vi "read station LIN config - 1.vi"(8 "error in":errorcluster, 10 "station idx":i32, 11 "configuration file path in":path) -> (0 "error out":errorcluster, 1 "LIN Device":T1={"Master Frame(3C)"="MasterReq\nSPA3414_ConfigurationsCMAGeely_CEMCALYPSOSDB34XX0Cfg_LIN3_190709_", "Slave Frame(3D)"="SlaveResp\nSPA3414_ConfigurationsCMAGeely_CEMCALYPSOSDB34XX0Cfg_LIN3_190709_", "Request Schedule"="CEMLIN3DiagRequestSchedule\nSPA3414_ConfigurationsCMAGeely_CEMCALYPSOSDB34XX0Cfg_LIN3_190709_", "Response Schedule"="CEMLIN3DiagResponseSchedule\nSPA3414_ConfigurationsCMAGeely_CEMCALYPSOSDB34XX0Cfg_LIN3_190709_", "Frame Write SCU"="", "Frame Read SCU"="", "LIN Name"=""}, 2 "LIN Device Name":string, 3 "configuration file path out":path)   [LabVIEW 2018]
uses:
  03.Inalfa LIN/LIN Device.ctl
  05.UserVI's/file io/ini/type defs/ini file actions.ctl
  05.UserVI's/file io/ini/type defs/ini entry value.ctl
  05.UserVI's/file io/ini/type defs/ini entry types.ctl
  05.UserVI's/file io/ini/type defs/ini entry.ctl
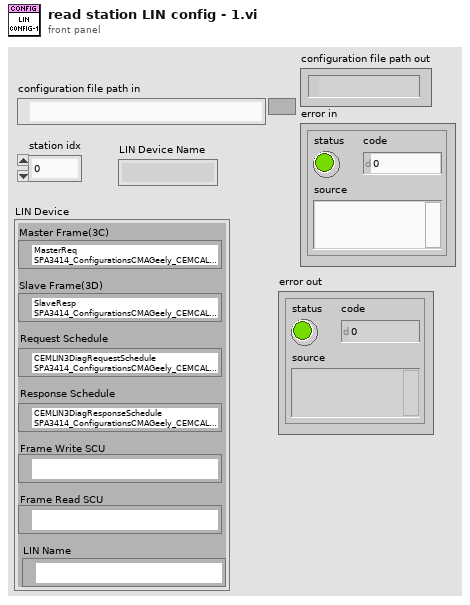
[diagram p1: front panel]
types:
  T1 = typedef "LIN Device.ctl" = cluster{"Master Frame(3C)":refnum<k21>, "Slave Frame(3D)":refnum<k21>, "Request Schedule":refnum<k21>, "Response Schedule":refnum<k21>, "Frame Write SCU":refnum<k21>, "Frame Read SCU":refnum<k21>, "LIN Name":refnum<k21>}
  T2 = typedef "ini entry value.ctl" = cluster{"Boolean":bool, "Dbl":dbl, "I32":i32, "Path":path, "String":string, "U32":u32}
  T3 = typedef "ini file actions.ctl" = enum16{"read ini", "write ini"}
  T4 = typedef "ini entry.ctl" = cluster{"section":string, "key":string, "type":T5, "default value":T2}
  T5 = typedef "ini entry types.ctl" = enum16{"Boolean", "Double", "I32", "Path", "String", "U32"}
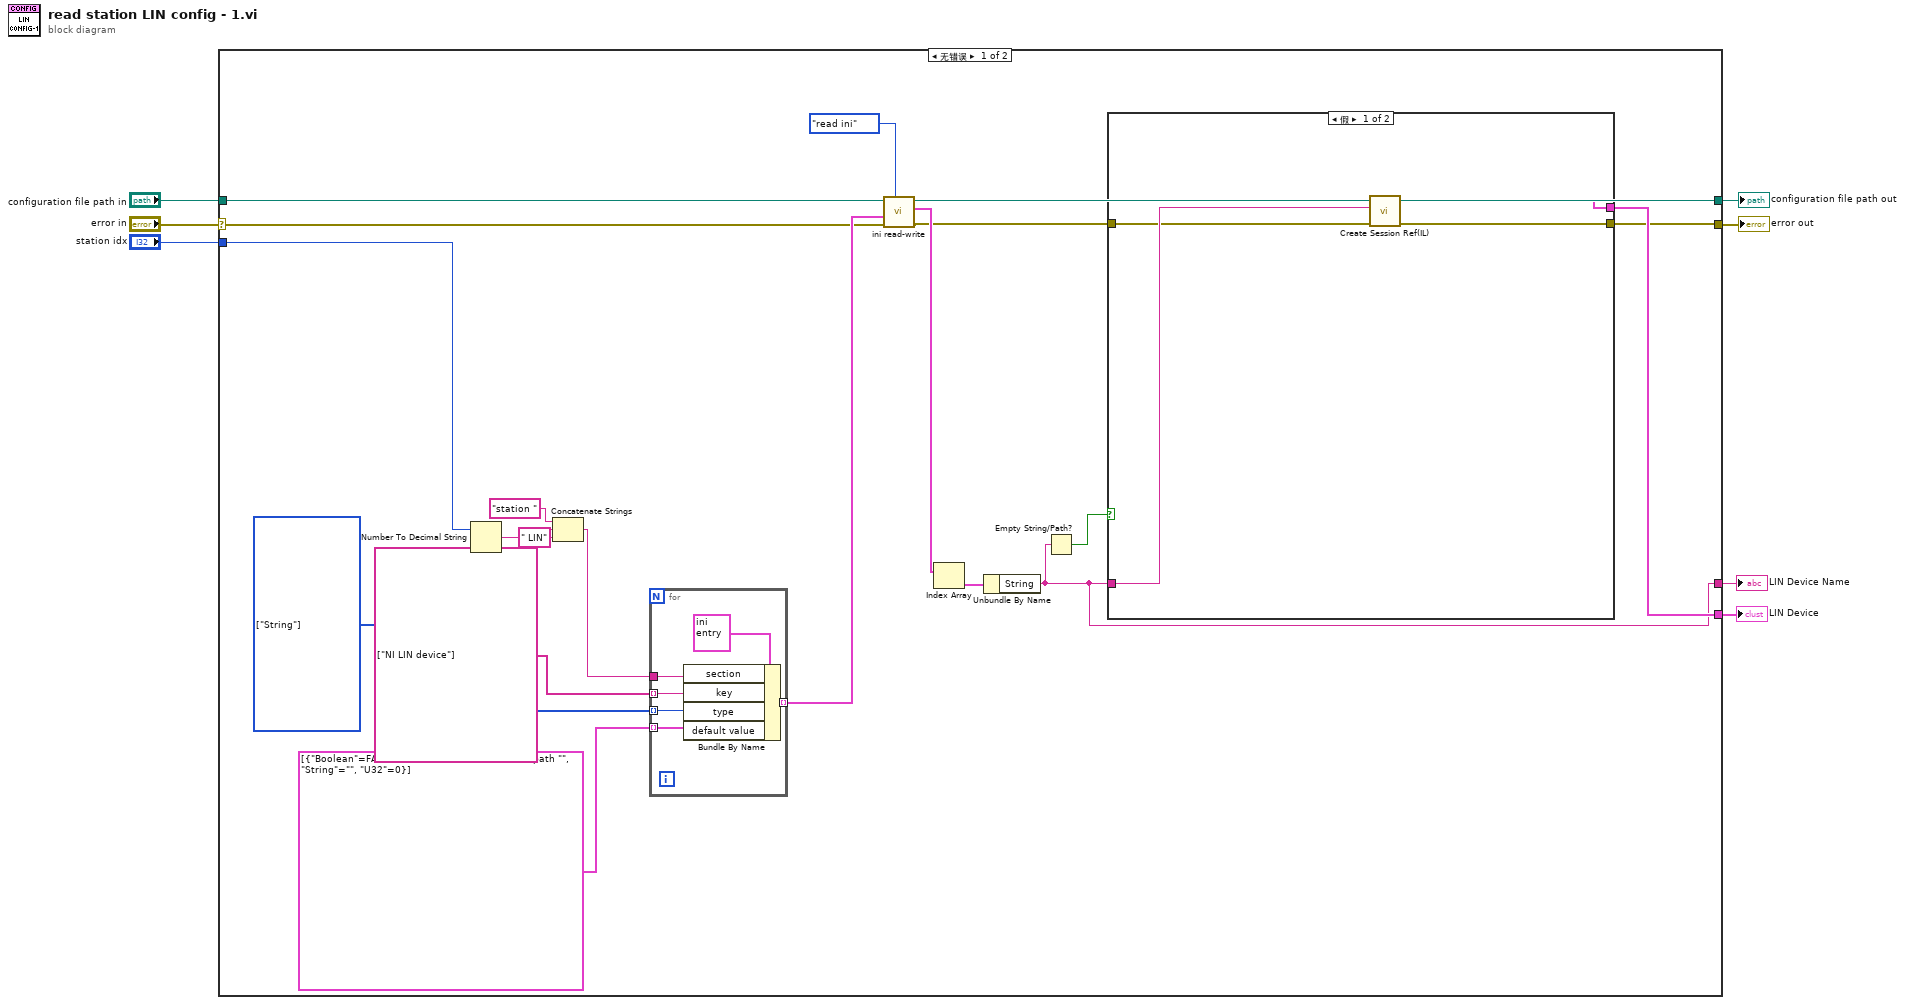
[diagram p0: block diagram]
diagram:
  n1 = case shown="无错误" "error in" {
    selector: "error in" -> [w15 w40]
    tunnel: "configuration file path in" -> [w27 w39]
    tunnel: [w24 w39] -> w6
    tunnel: [w10 w40] -> w5
    tunnel: "station idx" -> [w22 _]
    tunnel: [w9 _] -> w2
    tunnel: [w12 _] -> w1
    frame No Error {
      w18 = T5[] [enum."String"] items=["Boolean", "Double", "I32", "Path", "String", "U32"]
      n2 = Number To Decimal String(number=w22) -> (decimal integer string=w21:string)  [unwired: 1 in]
      n3 = Concatenate Strings("station ", w21, " LIN" ("string")) -> (w20:string)
      n4 = for {
        tunnel: w20 -> [w37]
        tunnel: string[] ["NI LIN device"] -> [w36] mode=indexing
        tunnel: w18 -> [w35] mode=indexing
        tunnel: T2[] [{"Boolean"=FALSE, "Dbl"=0.0, "I32"=0, "Path"=path "", "String"="", "U32"=0}] -> [w34] mode=indexing
        tunnel: [w33] -> w16 mode=indexing
        n5 = Bundle By Name(cluster=T4 {"section"="", "key"="", "type"=enum."Boolean", "default value"={"Boolean"=FALSE, "Dbl"=0.0, "I32"=0, "Path"=path "", "String"="", "U32"=0}}, "section"=w37, "key"=w36, "type"=w35, "default value"=w34) -> (w33:T4)
      }
      n6 = call "ini read-write.vi"("action"=ini_file_actions."read ini", "error in (no error)"=w15, "ini entry descriptors"=w16, "configuration file path"=w27) -> ("error out"=w11:errorcluster, "values out"=w25:T2[], "configuration file path out"=w24:path)  [unwired: 5 in]
      n7 = Index Array(array=w25) -> (element=w13:T2)  [unwired: 1 in]
      n8 = Unbundle By Name(w13) -> ("String"=w9:string)
      n9 = Empty String/Path?(string/path=w9) -> (empty?=w8:bool)
      n10 = case shown="假" w8 {
        tunnel: w9 -> [w31 _]
        tunnel: [w30 _] -> w12
        tunnel: w11 -> [w29 w32]
        tunnel: [w28 w32] -> w10
        frame False {
          n11 = call "Create Session Ref(IL).vi"("error in (no error)"=w29, "interface"=w31) -> ("error out"=w28:errorcluster, "LIN Device"=w30:T1)  [unwired: 8 in]
        }
        frame True {
        }
      }
    }
    frame Error {
    }
  }
  "configuration file path out" <- w6
  "error out" <- w5
  "LIN Device Name" <- w2
  "LIN Device" <- w1
